vi "Get Batch References.vi"(8 "error in (no error)":errorcluster, 10 "Control Names":string[](array[string]), 11 "Controls_Mgr in":refnum<class "Controls_Mgr.lvclass">) -> (0 "error out":errorcluster, 2 "Control References":refnum<vi>[](array[refnum]), 3 "Controls_Mgr out":refnum<class "Controls_Mgr.lvclass">)   [LabVIEW 2015, in "Generic Module Library.lvlib" / "Template G_Module.lvlib" / "Controls_Mgr.lvclass"]
uses:
  Controls_Mgr.lvclass
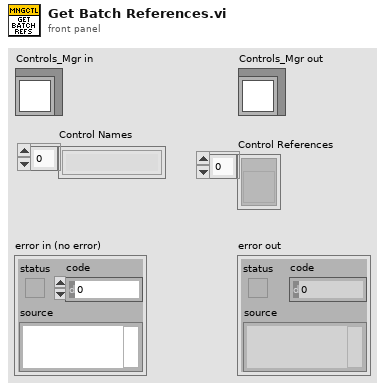
[diagram p1: front panel]
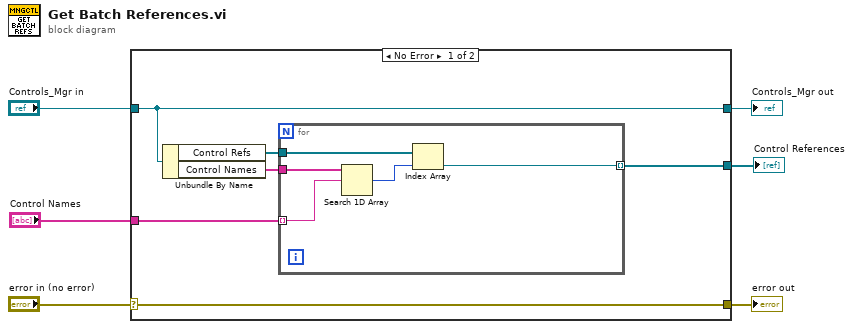
[diagram p0: block diagram]
diagram:
  n1 = case shown="No Error" "error in (no error)" {
    selector: "error in (no error)" -> [w12 w19]
    tunnel: [w12 w19] -> w5
    tunnel: [w10 w18] -> w3
    tunnel: "Controls_Mgr in" -> [w10 w18]
    tunnel: "Control Names" -> [w11 _]
    tunnel: [w7 _] -> w1
    frame No Error {
      n2 = Unbundle By Name(w10) -> ("Control Refs"=w8:refnum<vi>[], "Control Names"=w9:string[])
      n3 = for {
        tunnel: w11 -> [w16] mode=indexing
        tunnel: w9 -> [w17]
        tunnel: w8 -> [w15]
        tunnel: [w13] -> w7 mode=indexing
        n4 = Search 1D Array(1D array=w17, element=w16) -> (index of element=w14:i32)  [unwired: 1 in]
        n5 = Index Array(array=w15, index=w14) -> (element=w13:refnum<vi>)
      }
    }
    frame Error {
    }
  }
  "error out" <- w5
  "Controls_Mgr out" <- w3
  "Control References" <- w1
